vi "Get_RFID_Baseband.vi"(0 "input complex waveform":T1={"t0"=0.0, "dt"=1.0, "Y"=[]} {"Y" format="%.3f"; "dt" format="%^.2e"; "t0" format="%.4f"}) -> (4 "Recovered Waveform Graph":cluster{"t0":dbl, "dt":dbl, "Y":dbl[]}(graph), 6 "output bit stream":i8[](array[numeric]))   [LabVIEW 2015]
uses:
  <vilib>/addons/Modulation/Analog/controls/Complex Data Waveform.ctl
  <vilib>/addons/Modulation/Analog/support/mod_Set Error Source.vi
  <vilib>/addons/Modulation/Digital/General/MT Generate ASK system parameters (M).vi
  <vilib>/addons/Modulation/Digital/Support/Common/Validators/mod_Generate Filter Coefficients Validate.vi
  <vilib>/addons/Modulation/Digital/General/subVIs/mod_Generate Filter Coefficients.vi
  <vilib>/addons/Modulation/niDMT.lvlib
  <vilib>/addons/Modulation/niAMT.lvlib
panel:
  out "error out 2":errorcluster caption="error out"
  in  "error in":errorcluster
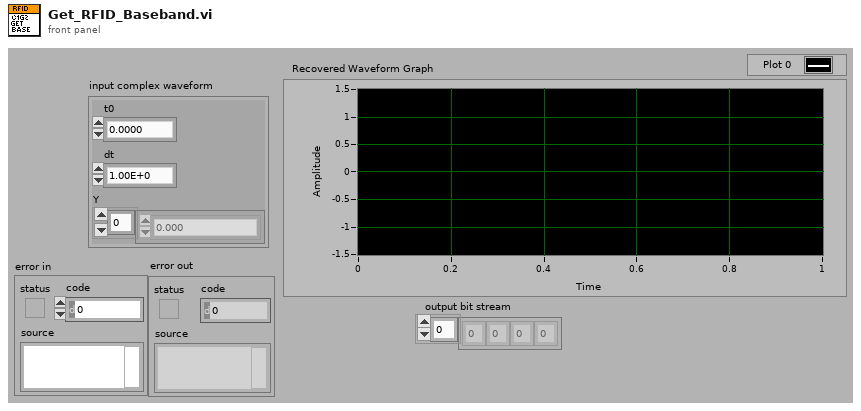
[diagram p1: front panel]
types:
  T1 = typedef "niAMT.lvlib/Complex Data Waveform.ctl" = cluster{"t0":dbl, "dt":dbl, "Y":cdb[]}
  T2 = enum16{"none", "Raised Cosine", "Root Raised Cos", "Gaussian"}
  T3 = cluster{"samples per symbol (16)":i32, "symbol map":cdb[]}
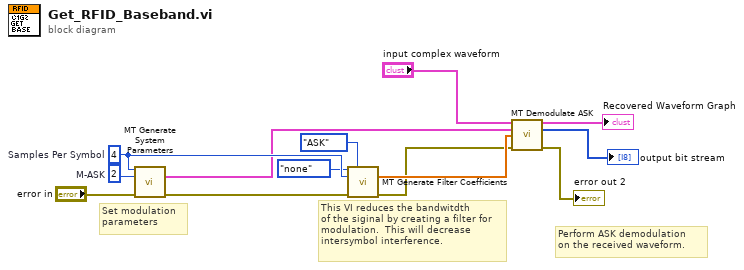
[diagram p0: block diagram]
diagram:
  w12 = 2  # M-ASK
  w9 = 4  # Samples Per Symbol
  # "Set modulation \nparameters"
  # "Perform ASK demodulation \non the received waveform."
  # "This VI reduces the bandwitdth\nof the siginal by creating a filter for\nmodulation.  This will decrease\nintersymbol interference."
  n1 = call-poly <vilib>:"MT Generate System Parameters.vi"("samples per symbol (16)"=w9, "M-ASK (2)"=w12, "error in (no error)"="error in") -> ("ASK system parameters"=w7:T3, "error out"=w10:errorcluster)  [unwired: 10 in, 1 out]
  n2 = call <vilib>:"MT Generate Filter Coefficients.vi"("pulse shaping filter (none)"=T2."none", "modulation type"=enum16{"FSK", "PSK", "QAM", "MSK", "PAM", "ASK"}."ASK", "pulse shaping samples per symbol (16)"=w9, "error in (no error)"=w10) -> ("matched filter coefficients"=w6:dbl[], "error out"=w4:errorcluster)  [unwired: 9 in, 1 out]
  n3 = call <vilib>:"MT Demodulate ASK.vi"("input complex waveform"="input complex waveform", "ASK system parameters"=w7, "matched filter coefficients"=w6, "error in (no error)"=w4) -> ("recovered complex waveform"=→"Recovered Waveform Graph":T1, "output bit stream"=→"output bit stream":i8[], "error out"=→"error out 2":errorcluster)  [unwired: 7 in, 2 out]
